vi "svmdense_save_model.vi"(8 "error in (no error)":errorcluster, 10 "Model":T1, 11 "Save path":path) -> (0 "error out":errorcluster)   [LabVIEW 2015]
uses:
  Controls/svmdense_model.ctl
  LibSVM Sparse/Wrapper API/Controls/svm_parameter.ctl
  LibSVM Sparse/Wrapper API/Controls/svm_type.ctl
  LibSVM Sparse/Wrapper API/Controls/svm_kernel_type.ctl
  bin/LabVIEW-libsvm-dense.so
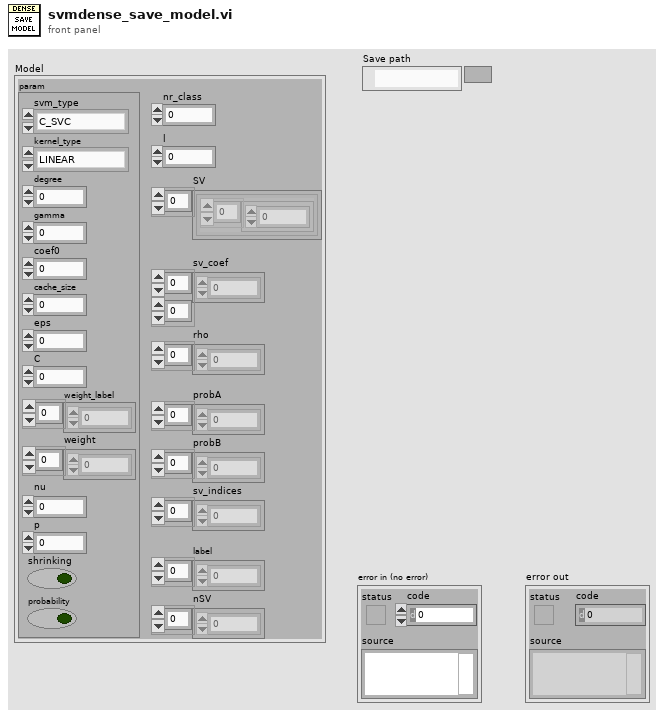
[diagram p1: front panel]
types:
  T1 = typedef "svmdense_model.ctl" = cluster{"param":T2, "nr_class":i32, "l":i32, "SV":cluster{"Array":dbl[]}[], "sv_coef":dbl[][], "rho":dbl[], "probA":dbl[], "probB":dbl[], "sv_indices":i32[], "label":i32[], "nSV":i32[]}
  T2 = typedef "svm_parameter.ctl" = cluster{"svm_type":T3, "kernel_type":T4, "degree":i32, "gamma":dbl, "coef0":dbl, "cache_size":dbl, "eps":dbl, "C":dbl, "weight_label":i32[], "weight":dbl[], "nu":dbl, "p":dbl, "shrinking":bool, "probability":bool}
  T3 = typedef "svm_type.ctl" = enum32{"C_SVC", "NU_SVC", "ONE_CLASS", "EPSILON_SVR", "NU_SVR"}
  T4 = typedef "svm_kernel_type.ctl" = enum32{"LINEAR", "POLY", "RBF", "SIGMOID", "PRECOMPUTED"}
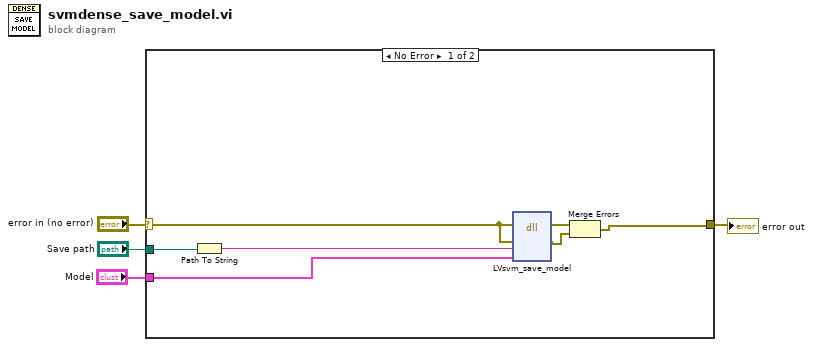
[diagram p0: block diagram]
diagram:
  n1 = case shown="No Error" "error in (no error)" {
    selector: "error in (no error)" -> [w9 w12]
    tunnel: [w8 w12] -> w4
    tunnel: "Save path" -> [w11 _]
    tunnel: "Model" -> [w7 _]
    frame No Error {
      n2 = Path To String(path=w11) -> (string=w10:string)
      n3 = dll-call lib="home/os/dev/LabVIEW-libsvm/LabVIEW/bin/LabVIEW-libsvm-dense.*" fn="LVsvm_save_model"(error in=w9, "lvErr"=w9, "path_in"=w10, "model_in"=w7) -> (error out=w6:errorcluster, "lvErr"=w5:errorcluster)  [unwired: 5 in, 1 out]
      n4 = Merge Errors(w6, w5) -> (w8:errorcluster)
    }
    frame Error {
    }
  }
  "error out" <- w4
